vi "Configure Dialog.vi"(8 "error in (no error)":errorcluster, 11 "Configure Operation Mode Msg in":refnum<class "Configure Operation Mode Msg.lvclass">) -> (0 "error out":errorcluster, 2 "Ok?":bool, 3 "Configure Operation Mode Msg out":refnum<class "Configure Operation Mode Msg.lvclass">)   [LabVIEW 2014, in "CS++Fgen.lvlib" / "Configure Operation Mode Msg.lvclass"]
uses:
  Configure Operation Mode Msg.lvclass
  CSPP_Core/Actors/CS++PVMonitor Messages/CS++PVUpdate Msg/CS++PVUpdate Msg.lvclass
panel:
  in  "Operation Mode":i32(ring) caption="operation mode (Continuous)" items=["Continuous", "Burst"]
  in  "channel name (\"CHANNEL1\")":string="CHANNEL1" caption="Channel Name"
  in  "OK Button":bool
  in  "Cancel Button":bool
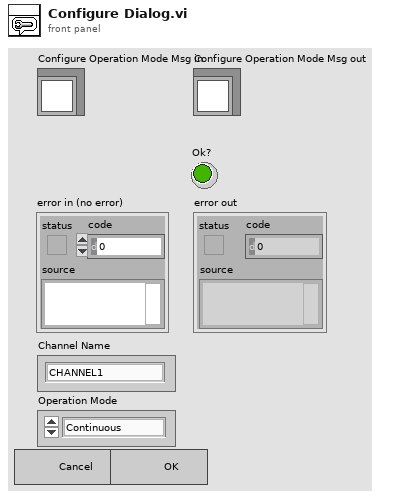
[diagram p1: front panel]
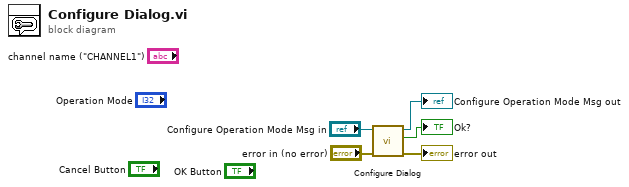
[diagram p0: block diagram]
diagram:
  n1 = call-parent "Configure Dialog.vi"("error in (no error)"="error in (no error)", "Message in"="Configure Operation Mode Msg in") -> ("error out"=→"error out":errorcluster, "Ok?"=→"Ok?":bool, "Message out"=→"Configure Operation Mode Msg out":refnum<class "Configure Operation Mode Msg.lvclass">)  [unwired: 7 in]
